vi "CTRE_ServoBlock_SmartTankStraightDistance.vi"(7 "Done Timeout":dbl, 10 "Timeout":dbl, 11 "Sensored Tank Servo Distance":T9) -> (0 "Reached Target":bool, 3 "Sensored Tank":T1={"Sensored Gearbox Left"={"Smart Motor Controller"={"DeviceStatus"={"status"=FALSE, "code"=0, "source"=""}, "Type"=enum."PWM", "PWM"={"PWM Channel"=enum."PWM 1", "DeadBand"={"Name"="", "maxPositivePwm"=0, "minPositivePwm"=0, "centerPwm"=0, "maxNegativePwm"=0, "minNegativePwm"=0, "angularRange"=0}}, "CAN"={"Device Number"=0, "SetOutput VI Ref"=variant(enum8{"Percent VBus", "Current", "Speed", "Position", "Voltage"} enum."Percent VBus"), "GetOutput VI Ref"=variant(refnum<k1> refnum), "Enable VI Ref"=variant(dbl 12.0), "Disable VI Ref"=variant(enum8{"Percent VBus", "Speed", "Position", "Slave", "Unchanged / Invalid", "Voltage Compensation", "Current", "Motion Profile"} enum."Percent VBus"), "Data"=variant}, "Invert"=FALSE}, "Invert"=FALSE, "Gear Ratio"=0.0}, "Sensored Gearbox Right "={"Smart Motor Controller"={"DeviceStatus"={"status"=FALSE, "code"=0, "source"=""}, "Type"=enum."PWM", "PWM"={"PWM Channel"=enum."PWM 1", "DeadBand"={"Name"="", "maxPositivePwm"=0, "minPositivePwm"=0, "centerPwm"=0, "maxNegativePwm"=0, "minNegativePwm"=0, "angularRange"=0}}, "CAN"={"Device Number"=0, "SetOutput VI Ref"=variant(enum8{"Percent VBus", "Current", "Speed", "Position", "Voltage"} enum."Percent VBus"), "GetOutput VI Ref"=variant(refnum<k1> refnum), "Enable VI Ref"=variant(dbl 12.0), "Disable VI Ref"=variant(enum8{"Percent VBus", "Speed", "Position", "Slave", "Unchanged / Invalid", "Voltage Compensation", "Current", "Motion Profile"} enum."Percent VBus"), "Data"=variant}, "Invert"=FALSE}, "Invert"=FALSE, "Gear Ratio"=0.0}, "Wheel Radius"=0.0, "Distance Between Wheels"=0.0})   [LabVIEW 2016]
uses:
  <vilib>/Rock Robotics/WPI/ThirdParty/CanMotor/CTRLib-LV-TalonSRX/Framework/SensoredTank.ctl
  <vilib>/Rock Robotics/WPI/ThirdParty/CanMotor/CTRLib-LV-TalonSRX/Framework/SensoredGearbox.ctl
  <vilib>/Rock Robotics/WPI/MotorControl/WPI_MotorControlDeviceRef.ctl
  <vilib>/Rock Robotics/WPI/MotorControl/WPI_MotorControlType.ctl
  <vilib>/Rock Robotics/SystemInterfaces/DIO/FPGA_DIOPWMChannel.ctl
  <vilib>/Rock Robotics/WPI/PWM/WPI_PWMDeadband.ctl
  <vilib>/Rock Robotics/WPI/ThirdParty/CanMotor/CTRLib-LV-TalonSRX/CTRE_CANTalonSRX_ControlMode.ctl
  <vilib>/Rock Robotics/WPI/ThirdParty/CanMotor/CTRLib-LV-TalonSRX/Framework/ServoParams.ctl
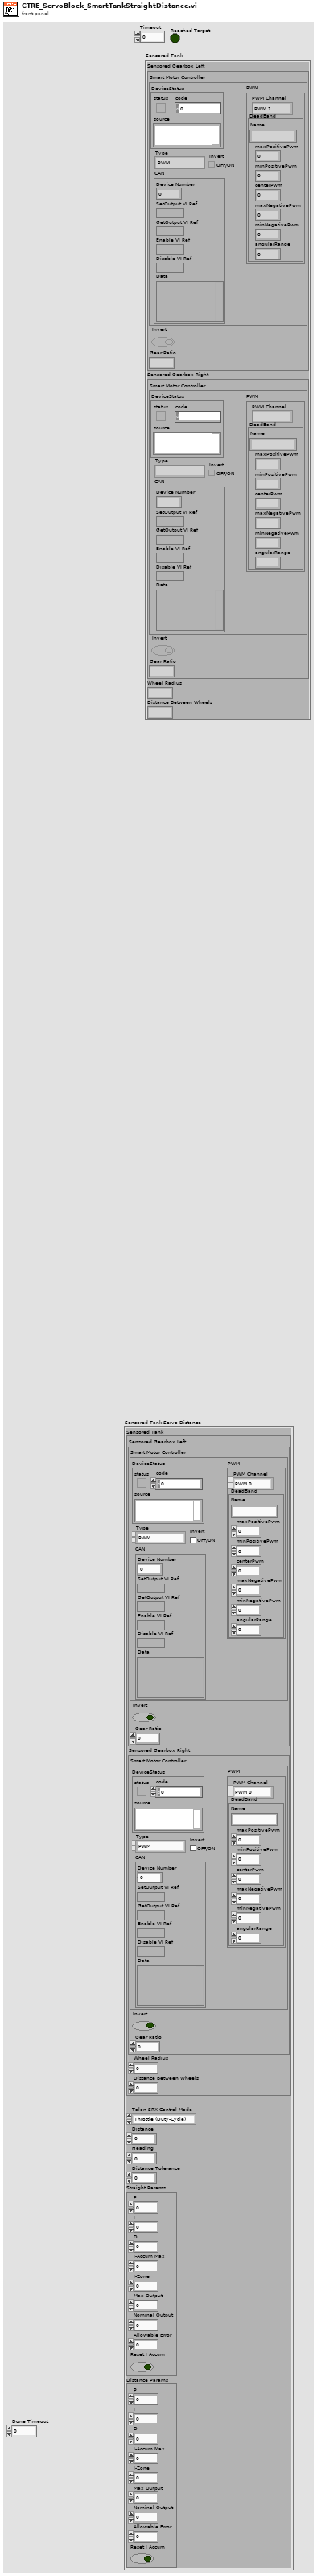
[diagram p1: front panel]
types:
  T1 = typedef "SensoredTank.ctl" = cluster{"Sensored Gearbox Left":T2, "Sensored Gearbox Right ":T2, "Wheel Radius":dbl, "Distance Between Wheels":dbl}
  T2 = typedef "SensoredGearbox.ctl" = cluster{"Smart Motor Controller":T3, "Invert":bool, "Gear Ratio":dbl}
  T3 = typedef "WPI_MotorControlDeviceRef.ctl" = cluster{"DeviceStatus":errorcluster, "Type":T4, "PWM":cluster{"PWM Channel":T5, "DeadBand":T6}, "CAN":cluster{"Device Number":u8, "SetOutput VI Ref":variant, "GetOutput VI Ref":variant, "Enable VI Ref":variant, "Disable VI Ref":variant, "Data":variant}, "Invert":bool}
  T4 = typedef "WPI_MotorControlType.ctl" = enum16{"PWM", "CAN"}
  T5 = typedef "FPGA_DIOPWMChannel.ctl" = enum8{"PWM 0", "PWM 1", "PWM 2", "PWM 3", "PWM 4", "PWM 5", "PWM 6", "PWM 7", "PWM 8", "PWM 9", "PWM MXP 0", "PWM MXP 1", "PWM MXP 2", "PWM MXP 3", "PWM MXP 4", "PWM MXP 5", "PWM MXP 6", "PWM MXP 7", "PWM MXP 8", "PWM MXP 9", "Invalid"}
  T6 = typedef "WPI_PWMDeadband.ctl" = cluster{"Name":string, "maxPositivePwm":i32, "minPositivePwm":i32, "centerPwm":i32, "maxNegativePwm":i32, "minNegativePwm":i32, "angularRange":u16}
  T7 = typedef "CTRE_CANTalonSRX_ControlMode.ctl" = enum16{"Throttle (Duty-Cycle)", "Position Closed-Loop", "Velocity Closed-Loop", "Current Closed-Loop", "Voltage Compensation", "Slave Follower", "Motion Profile", "Motion Magic"}
  T8 = typedef "ServoParams.ctl" = cluster{"P":dbl, "I":dbl, "D":dbl, "I-Accum Max":dbl, "I-Zone":dbl, "Max Output":dbl, "Nominal Output":dbl, "Allowable Error":dbl, "Reset I Accum":bool}
  T9 = cluster{"Sensored Tank":T1, "Talon SRX Control Mode":T7, "Distance":dbl, "Heading":dbl, "Distance Tolerance":dbl, "Straight Params":T8, "Distance Params":T8}
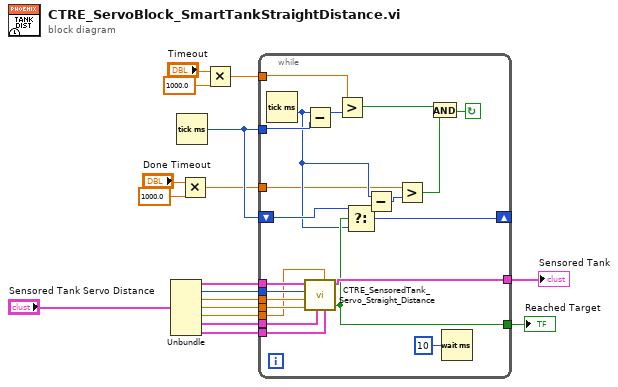
[diagram p0: block diagram]
diagram:
  n1 = Unbundle("Sensored Tank Servo Distance") -> ("Sensored Tank"=w17:T1, "Talon SRX Control Mode"=w16:T7, "Distance"=w15:dbl, "Heading"=w14:dbl, "Distance Tolerance"=w13:dbl, "Straight Params"=w12:T8, "Distance Params"=w11:T8)
  n2 = Tick Count (ms)() -> (millisecond timer value=w2:u32)
  n3 = Multiply(x="Done Timeout", y=1000.0) -> (x*y=w1:dbl)
  n4 = Multiply(x="Timeout", y=1000.0) -> (x*y=w8:dbl)
  n5 = while {
    tunnel: w17 -> [w38]
    tunnel: w16 -> [w37]
    tunnel: w15 -> [w36]
    tunnel: w14 -> [w35]
    tunnel: w13 -> [w34]
    tunnel: w12 -> [w33]
    tunnel: w11 -> [w32]
    tunnel: w2 -> [w31]
    tunnel: w8 -> [w29]
    tunnel: [w24] -> w7
    tunnel: [w25] -> w6
    shift-right: [w22] -> _
    shift-left: w2 -> [w23]
    tunnel: w1 -> [w19]
    stop <- w28 continue-if-true
    n6 = Tick Count (ms)() -> (millisecond timer value=w21:u32)
    n7 = Subtract(x=w21, y=w31) -> (x-y=w30:u32)
    n8 = call <vilib>:"CTRE_SensoredTank_Servo_Straight_Distance.vi"("Distance Params"=w32, "Distance Tolerance"=w34, "Straight Params"=w33, "Heading"=w35, "Distance"=w36, "Talon SRX Control Mode"=w37, "Sensored Tank"=w38) -> ("At Target"=w24:bool, "Sensored Tank"=w25:T1)  [unwired: 2 in, 1 out]
    n9 = Greater?(x=w29, y=w30) -> (0:w27:bool)
    n10 = Select(t=w23, s=w24, f=w21) -> (s? t:f=w22:u32)
    n11 = Subtract(x=w21, y=w22) -> (x-y=w20:u32)
    n12 = Greater?(x=w19, y=w20) -> (0:w18:bool)
    n13 = And(x=w27, y=w18) -> (x .and. y?=w28:bool)
    n14 = Wait (ms)(milliseconds to wait=u32 10) -> ()  [unwired: 1 out]
  }
  "Reached Target" <- w7
  "Sensored Tank" <- w6
